vi "Open.vi"(8 "error in (no error)":errorcluster, 11 "VisaResource in":refnum<class "VisaResource.lvclass">) -> (0 "error out":errorcluster, 3 "VisaResource out":refnum<class "VisaResource.lvclass">)   [LabVIEW 2020, in "PicoG-Core.lvlib" / "VisaResource.lvclass"]
uses:
  VisaResource.lvclass
  VisaResource.lvclass/VisaResource.ctl
  <vilib>/Instr/_visa.llb/VISA Configure Serial Port (Instr).vi
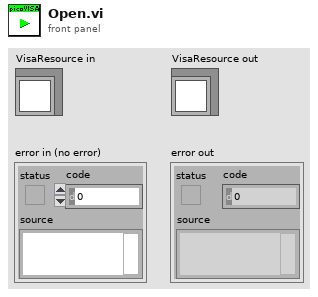
[diagram p1: front panel]
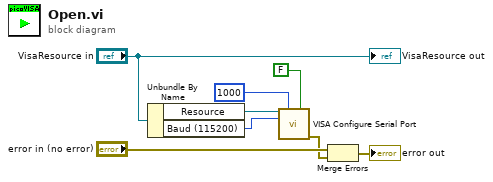
[diagram p0: block diagram]
diagram:
  n1 = Unbundle By Name("VisaResource in") -> ("Resource"=w6:refnum<visa-resource-name>, "Baud (115200)"=w5:u32)
  n2 = call-poly "VISA Configure Serial Port"("VISA resource name"=w6, "timeout (10sec)"=u32 1000, "Enable Termination\nChar (T)"=FALSE ("Enable Termination\nChar (T)"), "baud rate (9600)"=w5) -> ("error out"=w1:errorcluster)  [unwired: 10 in, 1 out]
  n3 = Merge Errors("error in (no error)", w1) -> (→"error out":errorcluster)
  "VisaResource out" <- "VisaResource in"
